vi "CRYSpiltOnlyUnit.vi"(10 "In Unit String":string) -> (2 "Out Unit String":string)   [LabVIEW 2013]
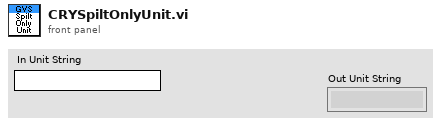
[diagram p1: front panel]
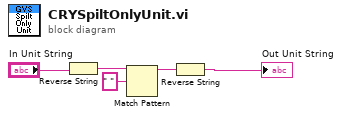
[diagram p0: block diagram]
diagram:
  n1 = Reverse String(1:"In Unit String") -> (0:w5:string)
  n2 = Match Pattern(string=w5, regular expression=" ") -> (before substring=w3:string)  [unwired: 1 in, 3 out]
  n3 = Reverse String(1:w3) -> (0:→"Out Unit String":string)
